vi "Array Manipulation.vi"() -> ()   [LabVIEW 2015]
doc: "This VI shows how different array functions can be used to manipulate data. There are also examples showing how we can use the Polymorphic functionality built into LabVIEW to easily modify the data in an array. \n\nExamine the different cases and read the comments on the block diagram for more details"
uses:
  <vilib>/measure/NI_MABase.lvlib
panel:
  in  "Stop Button":bool
  in  "Tab Control":T1(tab)
  out "Concatenated Data Array":dbl[](array[numeric])
  out "Concatenated Data":dbl[](graph)
  in  "Subtract?":bool
  out "Add or Subtract Data Array":dbl[](array[numeric])
  out "Add or Subtract Data":dbl[](graph)
  in  "Select Channel":u16(ring) items=["Channel 0", "Channel 1"]
  out "Single Channel of Data Array":dbl[](array[numeric])
  out "Single Channel of Data":dbl[](graph)
  out "Size of Array":i32
  in  "Offset":dbl(slide)=-8.326672684688674e-17 scale=-5.0..5.0
  out "Waveform Data":waveform(dbl)[](graph)
  out "Data Channel Array":dbl[][](array[numeric])
  in  "Channel 1 Offset":dbl(slide)=-8.326672684688674e-17 scale=-5.0..5.0
  out "All Data Channel":dbl[][](graph)
  out "Size of Array":i32[](array[numeric])
  out "Subset Data Array":dbl[][](array[numeric])
  in  "Start Value":i32(slide)=10 scale=0.0..1000.0
  out "Subset Data":dbl[][](graph)
  in  "Length":i32(slide)=1000 scale=0.0..1000.0
  # "Rows"
  # "Columns"
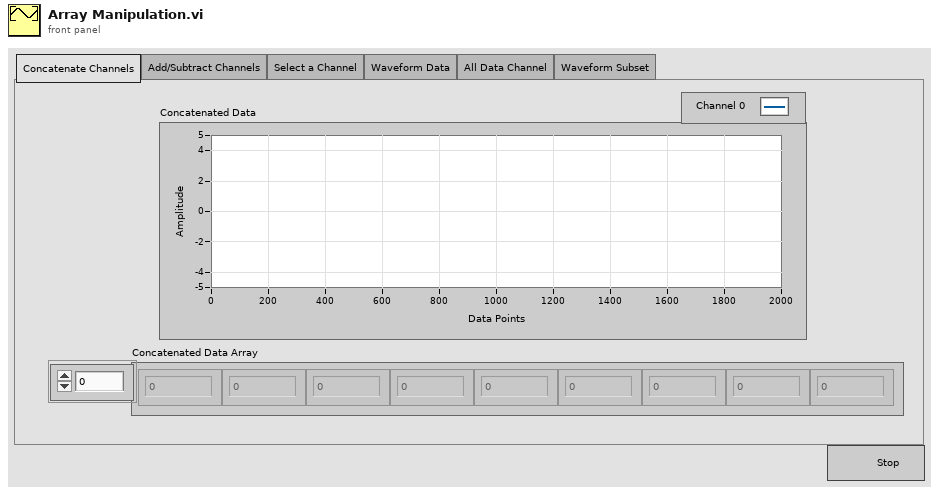
[diagram p1: front panel]
types:
  T1 = enum32{"Concatenate Channels", "Add/Subtract Channels", "Select a Channel", "Waveform Data", "All Data Channel", "Waveform Subset"}
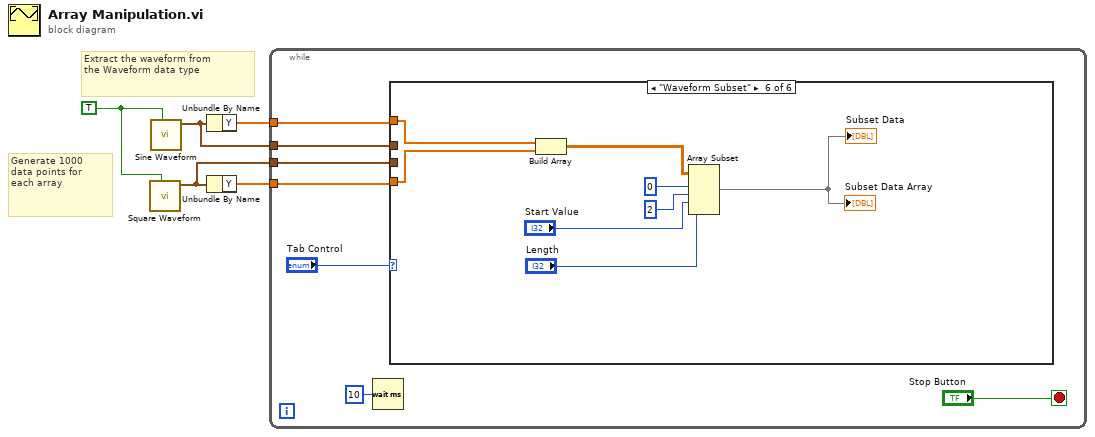
[diagram p0: block diagram]
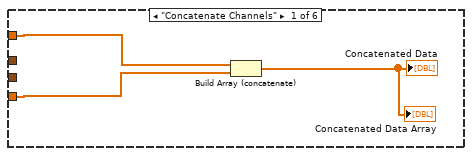
[diagram p2: hidden frame]
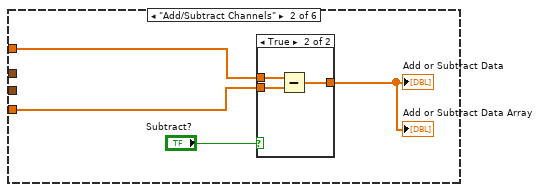
[diagram p3: hidden frame]
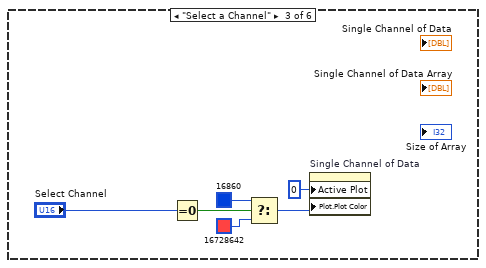
[diagram p5: hidden frame]
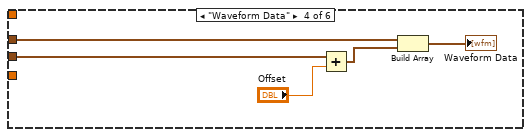
[diagram p6: hidden frame]
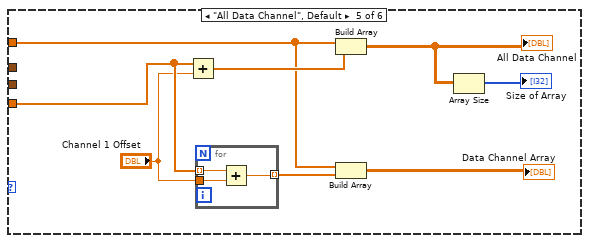
[diagram p7: hidden frame]
diagram:
  w5 = TRUE
  # "Extract the waveform from \nthe Waveform data type"
  # "Generate 1000\ndata points for \neach array"
  n1 = call <vilib>:"Square Waveform.vi"("reset signal"=w5) -> ("signal out"=w1:waveform(dbl))  [unwired: 9 in, 1 out]
  n2 = call <vilib>:"Sine Waveform.vi"("reset signal"=w5) -> ("signal out"=w2:waveform(dbl))  [unwired: 9 in, 1 out]
  n3 = Unbundle By Name(w2) -> ("Y"=w4:dbl[])
  n4 = Unbundle By Name(w1) -> ("Y"=w3:dbl[])
  n5 = while {
    tunnel: w4 -> [w10]
    tunnel: w3 -> [w9]
    tunnel: w2 -> [w8]
    tunnel: w1 -> [w7]
    stop <- "Stop Button" stop-if-true
    n6 = Wait (ms)(milliseconds to wait=u32 10) -> ()  [unwired: 1 out]
    n7 = case shown="\"Waveform Subset\"" "Tab Control" {
      tunnel: w10 -> [w14 w19 _ _ w38 w47]
      tunnel: w9 -> [w13 w18 _ _ w40 w46]
      tunnel: w8 -> [_ _ _ w30 _ _]
      tunnel: w7 -> [_ _ _ w32 _ _]
      frame "Concatenate Channels" {
        n8 = Build Array (concatenate)(w14, w13) -> (→"Concatenated Data" →"Concatenated Data Array":dbl[])
      }
      frame "Add/Subtract Channels" {
        n9 = case shown="True" "Subtract?" {
          tunnel: w19 -> [_ w22]
          tunnel: w18 -> [_ w21]
          tunnel: [_ w20] -> w16
          frame False {
          }
          frame True {
            n10 = Subtract(x=w22, y=w21) -> (x-y=w20:dbl[])
          }
        }
        "Add or Subtract Data" <- w16
        "Add or Subtract Data Array" <- w16
      }
      frame "Select a Channel" {
        n11 = Equal To 0?(x="Select Channel") -> (x = 0?=w24:bool)
        n12 = Select(t=u32 16860, s=w24, f=u32 16728642) -> (s? t:f=w27:u32)
        n13 = property on="Single Channel of Data" class="WFGraph (strict)"("Active Plot"=u32 0, "Plot.Plot Color"=w27) -> ()  [unwired: 2 in, 2 out]
      }
      frame "Waveform Data" {
        n14 = Add(x=w32, y="Offset") -> (x+y=w31:waveform(dbl))
        n15 = Build Array(w30, w31) -> (→"Waveform Data":waveform(dbl)[])
      }
      frame "All Data Channel", Default {
        n16 = Add(x=w40, y="Channel 1 Offset") -> (x+y=w41:dbl[])
        n17 = for {
          tunnel: w40 -> [w44] mode=indexing
          tunnel: "Channel 1 Offset" -> [w43]
          tunnel: [w42] -> w37 mode=indexing
          n18 = Add(x=w44, y=w43) -> (x+y=w42:dbl)
        }
        n19 = Build Array(w38, w41) -> (w36:dbl[][])
        "All Data Channel" <- w36
        n20 = Build Array(w38, w37) -> (→"Data Channel Array":dbl[][])
        n21 = Array Size(array=w36) -> (size(s)=→"Size of Array":i32[])
      }
      frame "Waveform Subset" {
        n22 = Build Array(w47, w46) -> (w48:dbl[][])
        n23 = Array Subset "Array Subset"(array=w48, index (row)=0 ("index"), length (row)=2 ("length"), index (col)="Start Value", length (col)="Length") -> (→"Subset Data Array" →"Subset Data":dbl[][])
      }
    }
  }
